vi "Write Expected Channel Count.vi"(8 "error in":errorcluster, 10 "expected channel count":i32, 11 "module test in":refnum<class "Module Test.lvclass">) -> (0 "error out":errorcluster, 3 "module test out":refnum<class "Module Test.lvclass">)   [LabVIEW 2020, in "Module Test.lvclass"]
uses:
  Module Test.lvclass
  Module Test.lvclass/Module Test.ctl
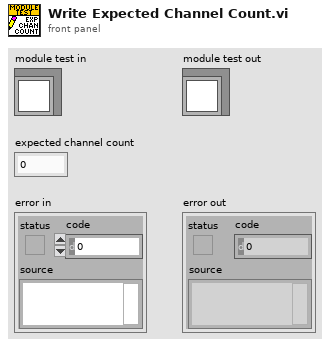
[diagram p1: front panel]
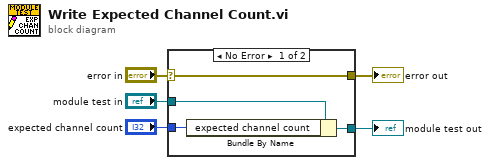
[diagram p0: block diagram]
diagram:
  n1 = case shown="No Error" "error in" {
    selector: "error in" -> [w9 w10]
    tunnel: [w9 w10] -> w4
    tunnel: [w7 w11] -> w2
    tunnel: "module test in" -> [w8 w11]
    tunnel: "expected channel count" -> [w6 _]
    frame No Error {
      n2 = Bundle By Name(cluster=w8, "expected channel count"=w6) -> (w7:refnum<class "Module Test.lvclass">)
    }
    frame Error {
    }
  }
  "error out" <- w4
  "module test out" <- w2
